vi "Simple Reader.vi"(8 "error in (no error)":errorcluster, 11 "ZI Lockin in":refnum<class "ZI Lockin.lvclass">) -> (0 "error out":errorcluster, 2 "Signals":dbl[](array[numeric]), 3 "ZI Lockin out":refnum<class "ZI Lockin.lvclass">)   [LabVIEW 2016, in "ZI Lockin.lvclass"]
uses:
  ZI Lockin.lvclass
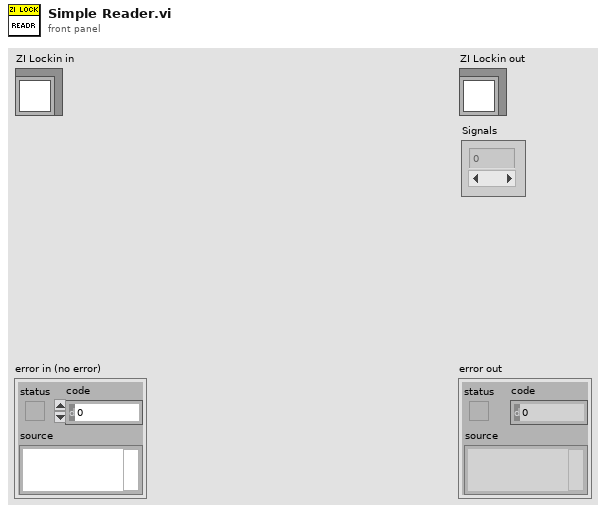
[diagram p1: front panel]
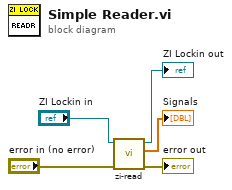
[diagram p0: block diagram]
diagram:
  n1 = call-dynamic "zi-read.vi"("error in (no error)"="error in (no error)", "ZI Lockin in"="ZI Lockin in") -> ("error out"=→"error out":errorcluster, "Result"=→"Signals":dbl[], "ZI Lockin out"=→"ZI Lockin out":refnum<class "ZI Lockin.lvclass">)  [unwired: 7 in]
